vi "NUMERIC TO STRING.vi"(5 "appended array":dbl[](array[numeric])) -> (2 "Array":string[](array[string]))   [LabVIEW 2017]
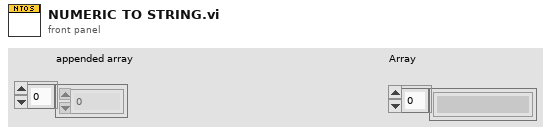
[diagram p1: front panel]
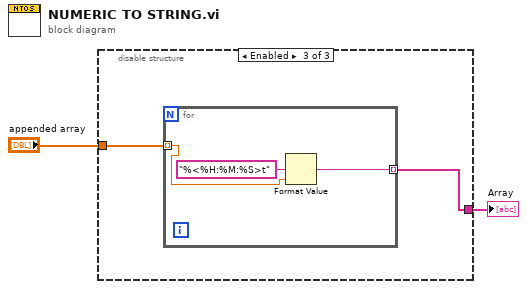
[diagram p0: block diagram]
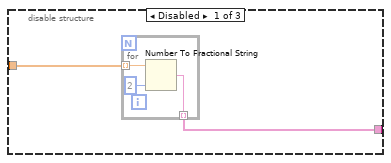
[diagram p2: hidden frame]
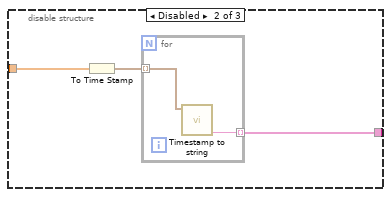
[diagram p3: hidden frame]
diagram:
  n1 = disable-structure shown="Enabled" {
    disable-tunnel: "appended array" -> [w4 w10 w14]
    disable-tunnel: [w3 w8 w13] -> w1
    frame Disabled {
      n2 = for {
        tunnel: w4 -> [w7] mode=indexing
        tunnel: [w6] -> w3 mode=indexing
        n3 = Number To Fractional String(number=w7, precision (6)=i16 2) -> (F-format string=w6:string)  [unwired: 2 in]
      }
    }
    frame Disabled {
      n4 = To Time Stamp(1:w10) -> (0:w9:timestamp[])
      n5 = for {
        tunnel: w9 -> [w12] mode=indexing
        tunnel: [w11] -> w8 mode=indexing
        n6 = call "Timestamp to string.vi"("time stamp"=w12) -> ("Time"=w11:string)  [unwired: 8 in, 2 out]
      }
    }
    frame Enabled {
      n7 = for {
        tunnel: w14 -> [w16] mode=indexing
        tunnel: [w15] -> w13 mode=indexing
        n8 = Format Value(format string="%<%H:%M:%S>t", value (0)=w16) -> (output string=w15:string)  [unwired: 1 in]
      }
    }
  }
  "Array" <- w1
